vi "LINX UART Read Benchmark.vi"() -> ()   [LabVIEW 2013]
uses:
  <vilib>/ptbypt/NI_PtbyPt.lvlib
  <vilib>/LabVIEW Hacker/LINX/LVH-LINX.lvlib
panel:
  in  "Stop Button":bool
  in  "Data":string
  out "Loop Rate":dbl(graph)
  out "Loop Time (ms)":i32
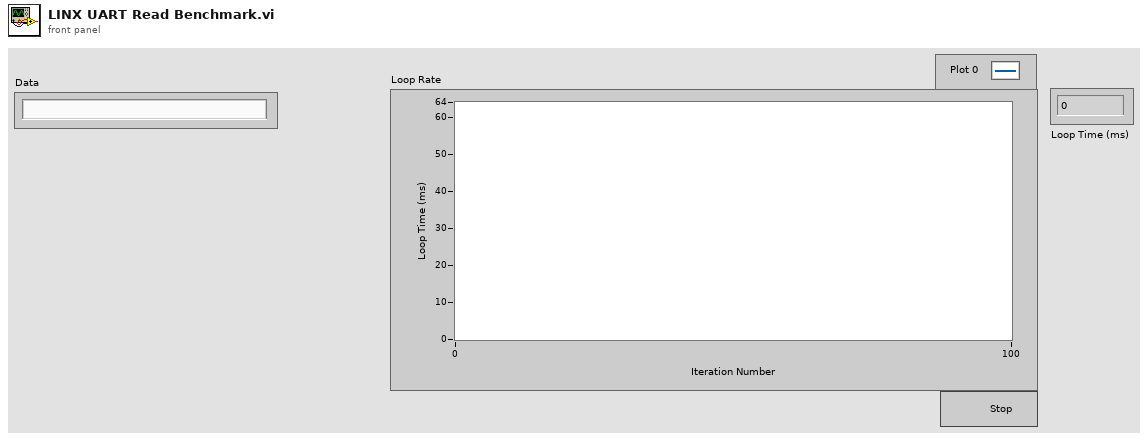
[diagram p1: front panel]
types:
  T1 = typedef "LVH-LINX.lvlib/LINX Ref.ctl" = cluster{"Platform":T2, "Interface":T3, "LINX Device Config":T4}
  T2 = typedef "LVH-LINX.lvlib/Platform.ctl" = enum16{"LINX", "myRIO"}
  T3 = typedef "LVH-LINX.lvlib/Interface.ctl" = enum16{"Serial", "TCP"}
  T4 = typedef "LVH-LINX.lvlib/Device.lvlib/LINX Device Config.ctl" = cluster{"Interface":T3, "COM Port":refnum<visa-resource-name>, "TCP Configuration":T5, "Device Family":T6, "Device ID":u8, "Device Name":string, "TCP Ref":refnum<k5>}
  T5 = typedef "LVH-LINX.lvlib/Device.lvlib/TCP Config.ctl" = cluster{"IP Address":string, "Port":u16}
  T6 = typedef "LVH-LINX.lvlib/Device Family.ctl" = enum8{"National Instruments", "Digilent", "Arduino"}
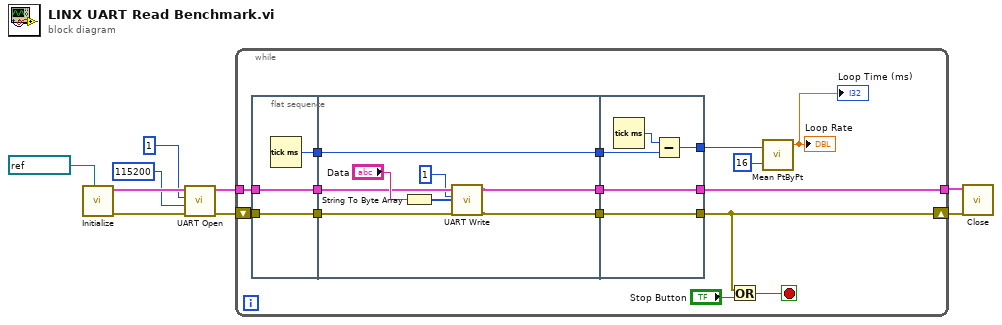
[diagram p0: block diagram]
diagram:
  n1 = call <vilib>:"Initialize.vi"("Serial Port"=refnum<visa-resource-name> "COM5" ("COM Port")) -> ("Error Out"=w7:errorcluster, "LINX Ref"=w8:T1)  [unwired: 8 in, 1 out]
  n2 = call <vilib>:"UART Open.vi"("Error In"=w7, "Baud Rate (9600)"=u32 115200, "UART Channel (0)"=u8 1 ("UART Channel"), "LINX Resource"=w8) -> ("Error Out"=w5:errorcluster, "LINX Resource"=w6:T1)  [unwired: 6 in]
  n3 = while {
    shift-right: [w10] -> w2
    shift-left: w5 -> [w17]
    tunnel: w6 -> [w13]
    tunnel: [w12] -> w1
    stop <- w24 stop-if-true
    n4 = flat-sequence {
      tunnel: [w27] -> w22
      tunnel: w17 -> [w26]
      tunnel: [w26] -> w16
      tunnel: [w25] -> w14
      tunnel: w13 -> [w25]
      tunnel: w22 -> [w35]
      tunnel: [w35] -> w21
      tunnel: w16 -> [w29]
      tunnel: [w33] -> w15
      tunnel: w14 -> [w30]
      tunnel: [w32] -> w11
      tunnel: w21 -> [w39]
      tunnel: [w38] -> w20
      tunnel: [w37] -> w10
      tunnel: w15 -> [w37]
      tunnel: [w36] -> w12
      tunnel: w11 -> [w36]
      frame #0 {
        n5 = Tick Count (ms)() -> (millisecond timer value=w27:u32)
      }
      frame #1 {
        n6 = String To Byte Array(string="Data") -> (unsigned byte array=w31:u8[])
        n7 = call <vilib>:"UART Write.vi"("Error In"=w29, "Data"=w31, "UART Channel (0)"=u8 1 ("UART Channel"), "LINX Resource"=w30) -> ("Error Out"=w33:errorcluster, "LINX Resource"=w32:T1)  [unwired: 6 in]
      }
      frame #2 {
        n8 = Tick Count (ms)() -> (millisecond timer value=w40:u32)
        n9 = Subtract(x=w40, y=w39) -> (x-y=w38:u32)
      }
    }
    n10 = Or(x=w10, y="Stop Button") -> (x .or. y?=w24:bool)
    n11 = call <vilib>:"Mean PtByPt.vi"("x"=w20, "sample length"=16) -> ("mean"=→"Loop Rate" →"Loop Time (ms)":dbl)  [unwired: 2 in, 1 out]
  }
  n12 = call <vilib>:"Close.vi"("Error In"=w2, "LINX Resource"=w1) -> ()  [unwired: 8 in, 2 out]
